vi "INTELLIFAUCET Temp Error Detect.vi"(8 "error in (no error)":errorcluster, 10 "Micro Amp":i32, 11 "Target":dbl) -> (0 "error out":errorcluster, 3 "Micro Amp Output":i32)   [LabVIEW 2019]
panel:
  out "Lower Limit":dbl
  out "Upper Limit":dbl
  out "Temp uA (Debug)":i32
  in  "Temp Debug":dbl
  out "?":dbl
  out "Temp (F)":dbl
  out "In Range?":bool
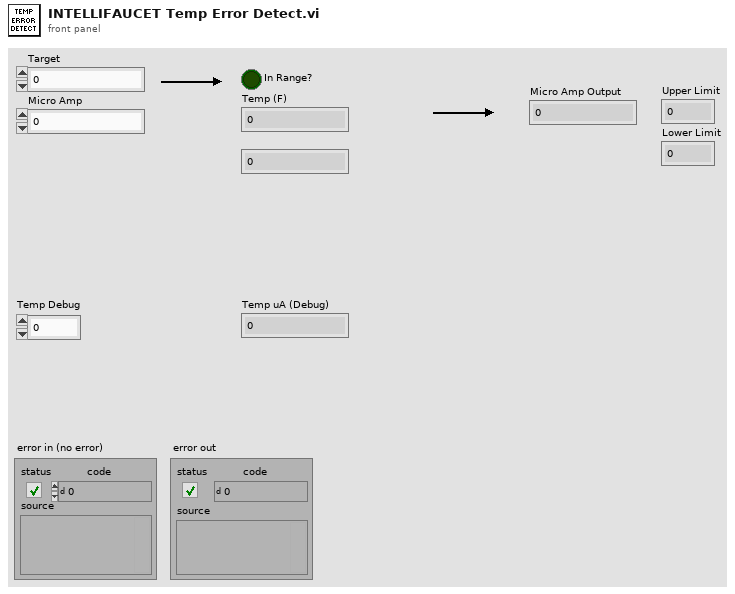
[diagram p1: front panel]
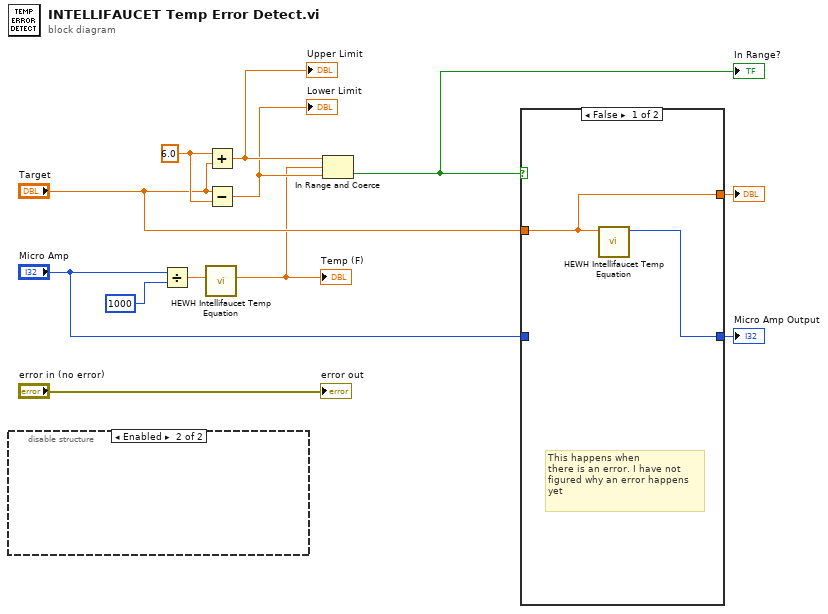
[diagram p0: block diagram]
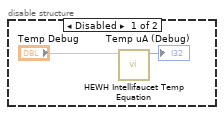
[diagram p2: hidden frame]
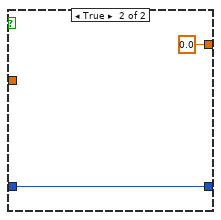
[diagram p3: hidden frame]
diagram:
  w12 = 6.0 ("x")
  n1 = disable-structure shown="Enabled" {
    frame Disabled {
      n2 = call "HEWH Intellifaucet Temp Equation.vi"("Temp/GPM Target"="Temp Debug") -> ("Temp uA"=→"Temp uA (Debug)":i32)  [unwired: 8 in, 2 out]
    }
    frame Enabled {
    }
  }
  n3 = Divide(x="Micro Amp", y=1000) -> (x/y=w11:dbl)
  n4 = call "HEWH Intellifaucet Temp Equation.vi"("mA to F"=w11) -> ("Temp (F)"=w2:dbl)  [unwired: 8 in, 2 out]
  "Temp (F)" <- w2
  n5 = Add(x=w12, y="Target") -> (x+y=w4:dbl)
  "Upper Limit" <- w4
  n6 = Subtract(x="Target", y=w12) -> (x-y=w3:dbl)
  "Lower Limit" <- w3
  n7 = In Range and Coerce(upper limit=w4, x=w2, lower limit=w3) -> (In Range?=w1:bool)  [unwired: 1 out]
  "In Range?" <- w1
  n8 = case shown="False" w1 {
    tunnel: "Micro Amp" -> [_ w18]
    tunnel: [w16 w18] -> w7
    tunnel: "Target" -> [w15 _]
    tunnel: [w15 0.0 ("Target")] -> w5
    frame False {
      # "This happens when\nthere is an error. I have not \nfigured why an error happens\nyet"
      n9 = call "HEWH Intellifaucet Temp Equation.vi"("Temp/GPM Target"=w15) -> ("Temp uA"=w16:i32)  [unwired: 8 in, 2 out]
    }
    frame True {
    }
  }
  "Micro Amp Output" <- w7
  "?" <- w5
  "error out" <- "error in (no error)"
